vi "Init GPIO Resources.vi"(8 "error in (no error)":errorcluster, 11 "Session in":refnum<class "Session.lvclass">) -> (0 "error out":errorcluster, 3 "Session out":refnum<class "Session.lvclass">)   [LabVIEW 2024, in "CTI.lvlib" / "Session.lvclass"]
uses:
  Session.lvclass
  GPIO Number.ctl
  GPIO/GPIO.lvclass
  Session.lvclass/Session.ctl
  CTI.lvlib
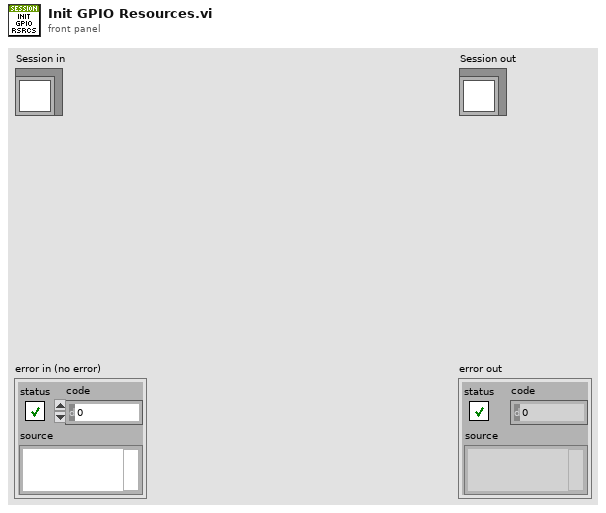
[diagram p1: front panel]
types:
  T1 = typedef "CTI.lvlib/GPIO Number.ctl" = i8
  T2 = typedef "CTI.lvlib/Session.lvclass/Resources.ctl" = cluster{"GPIO":map{T1, refnum<class "GPIO.lvclass">}, "AI":map{T3, refnum<class "AI.lvclass">}, "PWM":map{T1, refnum<class "PWM.lvclass">}, "UART":map{T4, refnum<class "UART.lvclass">}, "I2C":map{T5, refnum<class "I2C.lvclass">}, "SPI":map{T6, refnum<class "SPI.lvclass">}, "SPI CS":map{T1, refnum<class "SPI CS.lvclass">}}
  T3 = typedef "CTI.lvlib/ADC Number.ctl" = i8
  T4 = typedef "CTI.lvlib/UART Number.ctl" = i8
  T5 = typedef "CTI.lvlib/I2C Number.ctl" = i8
  T6 = typedef "CTI.lvlib/SPI Number.ctl" = i8
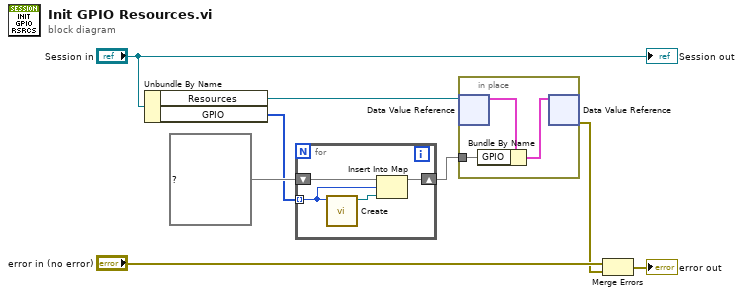
[diagram p0: block diagram]
diagram:
  n1 = Unbundle By Name("Session in") -> ("Resources"=w2:refnum<data-value>, "GPIO"=w3:u8[])
  n2 = for {
    tunnel: w3 -> [w11] mode=indexing
    shift-right: [w9] -> w5
    shift-left: map{T1, refnum<class "GPIO.lvclass">} {} ("GPIO") -> [w12]
    n3 = call "Create.vi"("GPIO #"=w11) -> ("GPIO out"=w10:refnum<class "GPIO.lvclass">)  [unwired: 9 in, 1 out]
    n4 = Insert Into Map(map in=w12, key=w11, value=w10) -> (map out=w9:map{T1, refnum<class "GPIO.lvclass">})  [unwired: 2 out]
  }
  n5 = in-place {
    in-place-border: w5 -> [w14]
    n6 = in-place-dvr #1(w2) -> (w15:T2)  [unwired: 1 out]
    n7 = Bundle By Name(cluster=w15, "GPIO"=w14) -> (w13:T2)
    n8 = in-place-dvr #1(w13) -> (w1:errorcluster)  [unwired: 1 out]
  }
  n9 = Merge Errors("error in (no error)", w1) -> (→"error out":errorcluster)
  "Session out" <- "Session in"
